vi "Noise-Create (Brickwall Filter).vi"(0 "Min Frequency (Hz)":dbl, 1 "Slope (dB/oct)":dbl, 2 "Slope Fmin (Hz)":dbl, 5 "Max Frequency (Hz)":dbl, 7 "Sampling rate (Hz)":dbl, 9 "Length (points)":i32, 11 "error in (no error)":errorcluster) -> (4 "Filtered Noise":dbl[](array[numeric]), 8 "dB Vrms of spectrum level = 0":dbl, 15 "error out":errorcluster)   [LabVIEW 2015]
uses:
  Utility VIs/Math VIs/LinSpace (x0-dx-npts).vi
  Noise-Globals.vi
  Utility VIs/Math VIs/dB to Linear (1D).vi
  Utility VIs/Math VIs/Linear to dB (scalar).vi
  Utility VIs/Math VIs/FFT x(t) to dB,Degrees (1D).vi
  <vilib>/Analysis/NI_AALBase.lvlib
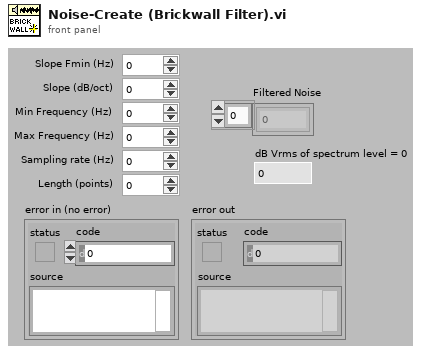
[diagram p1: front panel]
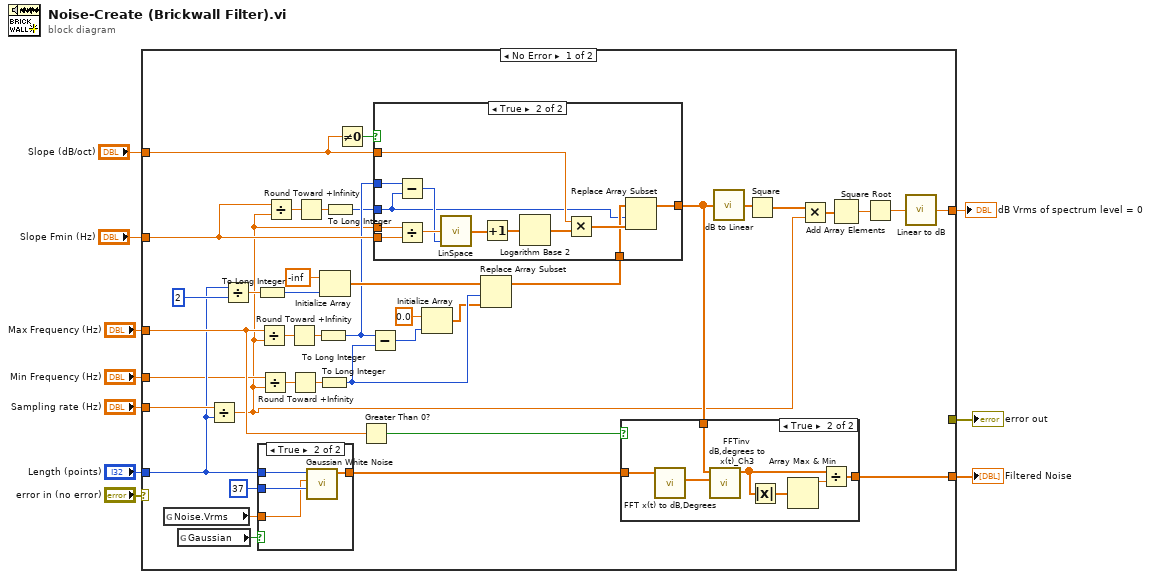
[diagram p0: block diagram]
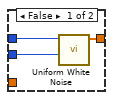
[diagram p3: hidden frame]
diagram:
  n1 = case shown="No Error" "error in (no error)" {
    selector: "error in (no error)" -> [_ w79]
    tunnel: [_ w79] -> w9
    tunnel: [w49 _] -> w4
    tunnel: "Max Frequency (Hz)" -> [w37 _]
    tunnel: "Min Frequency (Hz)" -> [w30 _]
    tunnel: "Sampling rate (Hz)" -> [w42 _]
    tunnel: "Length (points)" -> [w34 _]
    tunnel: "Slope (dB/oct)" -> [w28 _]
    tunnel: "Slope Fmin (Hz)" -> [w23 _]
    tunnel: [w16 _] -> w1
    frame No Error {
      n2 = global read "Noise-Globals.vi" "Noise.Vrms"() -> (w32:dbl)
      n3 = global read "Noise-Globals.vi" "Gaussian"() -> (w36:bool)
      n4 = Divide(x=w42, y=w34) -> (x/y=w15:dbl)
      n5 = Divide(x=w34, y=2) -> (x/y=w41:dbl)
      n6 = To Long Integer(number=w41) -> (32bit integer=w39:i32)
      n7 = case shown="True" w36 {
        tunnel: [w66 w70] -> w33
        tunnel: w34 -> [w65 w69]
        tunnel: 37 ("seed") -> [w64 w68]
        tunnel: w32 -> [_ w67]
        frame False {
          n8 = call <vilib>:"Uniform White Noise.vi"("seed"=w64, "samples"=w65) -> ("uniform white noise"=w66:dbl[])  [unwired: 8 in, 1 out]
        }
        frame True {
          n9 = call <vilib>:"Gaussian White Noise.vi"("seed"=w68, "standard deviation"=w67, "samples"=w69) -> ("Gaussian noise pattern"=w70:dbl[])  [unwired: 7 in, 1 out]
        }
      }
      n10 = Divide(x=w37, y=w15) -> (x/y=w44:dbl)
      n11 = Divide(x=w30, y=w15) -> (x/y=w46:dbl)
      n12 = Divide(x=w23, y=w15) -> (x/y=w24:dbl)
      n13 = Round Toward +Infinity(x=w44) -> (ceil(x): smallest int >= x=w45:dbl)
      n14 = Round Toward +Infinity(x=w46) -> (ceil(x): smallest int >= x=w47:dbl)
      n15 = Round Toward +Infinity(x=w24) -> (ceil(x): smallest int >= x=w25:dbl)
      n16 = To Long Integer(number=w45) -> (32bit integer=w22:i32)
      n17 = To Long Integer(number=w47) -> (32bit integer=w31:i32)
      n18 = Initialize Array(-inf ("element"), w39) -> (w43:dbl[])
      n19 = To Long Integer(number=w25) -> (32bit integer=w21:i32)
      n20 = Not Equal To 0?(x=w28) -> (x != 0?=w29:bool)
      n21 = Greater Than 0?(x=w37) -> (x > 0?=w38:bool)
      n22 = Subtract(x=w22, y=w31) -> (x-y=w26:i32)
      n23 = Initialize Array(0.0 ("element"), w26) -> (w20:dbl[])
      n24 = Replace Array Subset(array=w43, new element=w20, index=w31) -> (w19:dbl[])
      n25 = case shown="True" w29 {
        tunnel: w15 -> [_ w63]
        tunnel: w28 -> [_ w58]
        tunnel: [w50 w51] -> w18
        tunnel: w23 -> [_ w57]
        tunnel: w22 -> [_ w56]
        tunnel: w21 -> [_ w52]
        tunnel: w19 -> [w50 w53]
        frame False {
        }
        frame True {
          n26 = Subtract(x=w56, y=w52) -> (x-y=w55:i32)
          n27 = Divide(x=w63, y=w57) -> (x/y=w62:dbl)
          n28 = call-poly "LinSpace.vi"("npts"=w55, "dx"=w62) -> ("Array"=w61:dbl[])  [unwired: 2 in, 1 out]
          n29 = Increment(x=w61) -> (x+1=w60:dbl[])
          n30 = Logarithm Base 2(1:w60) -> (0:w59:dbl[])
          n31 = Multiply(x=w58, y=w59) -> (x*y=w54:dbl[])
          n32 = Replace Array Subset(array=w53, new element=w54, index=w52) -> (w51:dbl[])
        }
      }
      n33 = case shown="True" w38 {
        tunnel: w33 -> [w71 w75]
        tunnel: [w71 w74] -> w49
        tunnel: w18 -> [_ w73]
        frame False {
        }
        frame True {
          n34 = call-poly "FFT x(t) to dB,Degrees.vi"("X"=w75) -> ("+Freq Phase of FFT (degrees)"=w72:dbl[])  [unwired: 8 in, 2 out]
          n35 = call "FFTinv dB,degrees to x(t)_Ch3.vi"("+Freq Phase of FFT (degrees)"=w72, "+Freq. Mag of FFT (rms dB)"=w73) -> ("X(t)"=w76:dbl[])  [unwired: 8 in, 1 out]
          n36 = Absolute Value(x=w76) -> (abs(x)=w78:dbl[])
          n37 = Array Max & Min(array=w78) -> (max value=w77:dbl)  [unwired: 3 out]
          n38 = Divide(x=w76, y=w77) -> (x/y=w74:dbl[])
        }
      }
      n39 = call-poly "dB to Linear.vi"("dB"=w18) -> ("linear"=w14:dbl[])
      n40 = Square(x=w14) -> (x^2=w11:dbl[])
      n41 = Multiply(x=w11, y=w15) -> (x*y=w12:dbl[])
      n42 = Add Array Elements(numeric array=w12) -> (sum=w13:dbl)
      n43 = Square Root(x=w13) -> (sqrt(x)=w17:dbl)
      n44 = call-poly "Linear to dB.vi"("Linear"=w17) -> ("dB"=w16:dbl)
    }
    frame Error {
    }
  }
  "error out" <- w9
  "Filtered Noise" <- w4
  "dB Vrms of spectrum level = 0" <- w1
